vi "User Input Scanning Tank Size.vi"(3 "Height (mm)":dbl, 4 "Width (mm)":dbl, 5 "Length (mm)":dbl) -> (0 "Z Steps":string, 1 "Y Steps":string, 2 "X Steps":string)   [LabVIEW 2020]
doc: "Groups the individual X,Y,Z distance to step conversion into one sub-vi for the purpose of calculating the total number of steps to move the length,width and height of the scanning tank.\n\nArgs:\n\nLength (mm) Length of the scanning tank in the form of an integer\nWidth (mm): Width of the scanning tank in the form of an integer\nHeight (mm): Height of the scanning tank in the form of an integer\n\nReturns:\n\nX Steps: Number of steps required to go along the entire length of the scanning tank in the form of a string\nY Steps: Number of steps required to go along the entire width of the scanning tank in the form of a string\nZ Steps: Number of steps required to go along the entire height of the scanning tank in the form of a string"
panel:
  # "Width"
  # "Length"
  # "Height"
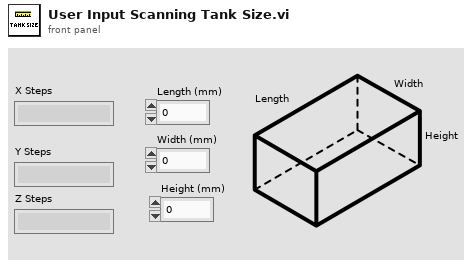
[diagram p1: front panel]
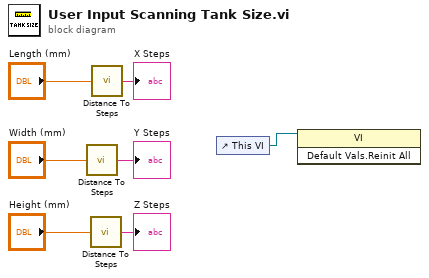
[diagram p0: block diagram]
diagram:
  n1 = call "Distance To Steps.vi"("Desired Distance (mm)"="Width (mm)") -> ("Number of Steps"=→"Y Steps":string)
  n2 = call "Distance To Steps.vi"("Desired Distance (mm)"="Height (mm)") -> ("Number of Steps"=→"Z Steps":string)
  n3 = call "Distance To Steps.vi"("Desired Distance (mm)"="Length (mm)") -> ("Number of Steps"=→"X Steps":string)
  n4 = control-ref of="This VI"() -> (w1:refnum<vi>)
  n5 = invoke class="VI" method="Default Vals.Reinit All"(reference=w1) -> ()  [unwired: 2 in, 3 out]
